vi "FSF_Query.vi"(0 "System no.":i32=1 min=1 max=4 step=1, 2 "Axes to query":string[](array[string]), 3 "All axes?":bool, 4 "Axis identifier?":bool, 5 "error in":errorcluster) -> (14 "Force value 1":dbl[](array[numeric]) format="%.6f", 15 "Position offset":dbl[](array[numeric]) format="%.6f", 16 "Force value 2":dbl[](array[numeric]) format="%.6f", 19 "error out":errorcluster)   [LabVIEW 2020]
doc: "Returns parameters used for last find surface procedure (FSF).\n\nC-413:"
panel:
  # "Returns the parameters set by FSF."
  # "If all axes: use"
  # "Query"
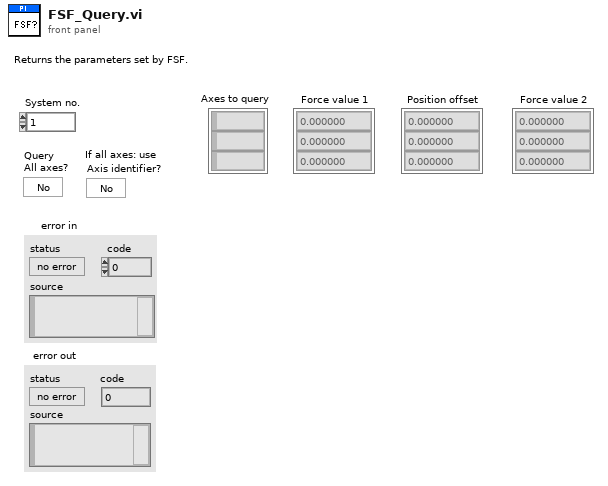
[diagram p1: front panel]
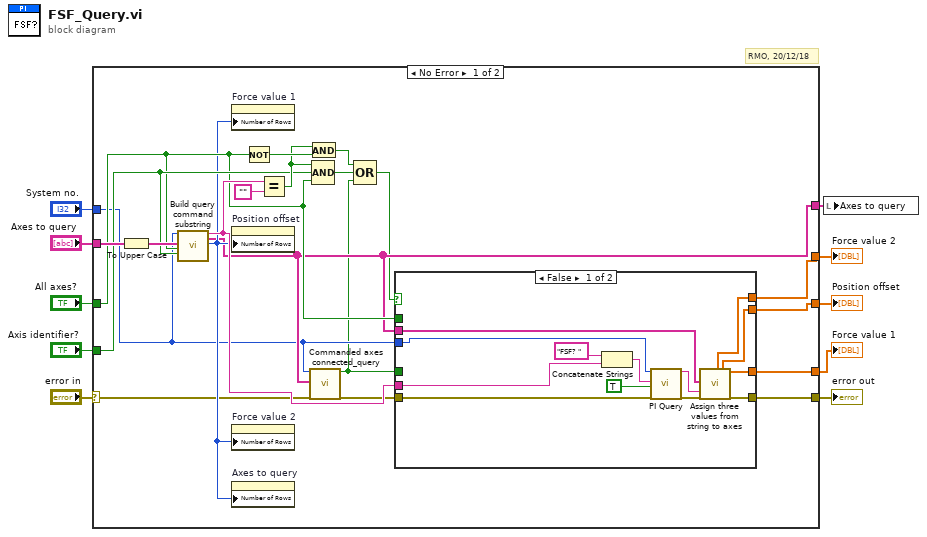
[diagram p0: block diagram]
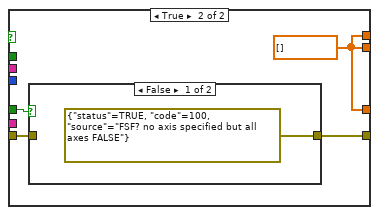
[diagram p2: hidden frame]
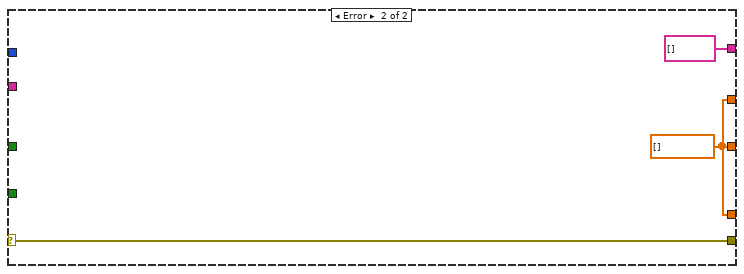
[diagram p4: hidden frame]
diagram:
  # "RMO, 20/12/18"
  n1 = case shown="No Error" "error in" {
    selector: "error in" -> [w11 w51]
    tunnel: [w31 w52] -> w10
    tunnel: "Axes to query" -> [w30 _]
    tunnel: [w22 w51] -> w8
    tunnel: "System no." -> [w16 _]
    tunnel: [w17 string[] [] ("Axes to query out")] -> w6
    tunnel: "Axis identifier?" -> [w24 _]
    tunnel: "All axes?" -> [w23 _]
    tunnel: [w21 w52] -> w3
    tunnel: [w20 w52] -> w2
    frame No Error {
      n2 = To Upper Case(1:w30) -> (0:w28:string[])
      n3 = call "Build query command substring.vi"("System no."=w16, "Axes to query in"=w28, "Query\nAll axes?"=w23, "For all axes: use\nAxis identifier?"=w24) -> ("Command substring"=w27:string, "Axes to query out"=w17:string[], "Number of rows"=w19:u32)  [unwired: 2 in, 11 out]
      n4 = property on="Force value 1" class="Arr (strict)"("Number of Rows"=w19) -> ()  [unwired: 2 in, 2 out]
      n5 = property on="Position offset" class="Arr (strict)"("Number of Rows"=w19) -> ()  [unwired: 2 in, 2 out]
      n6 = property on="Force value 2" class="Arr (strict)"("Number of Rows"=w19) -> ()  [unwired: 2 in, 2 out]
      n7 = property on="Axes to query" class="Arr (strict)"("Number of Rows"=w19) -> ()  [unwired: 2 in, 2 out]
      n8 = Not(x=w23) -> (.not. x?=w26:bool)
      n9 = Equal?(x=w27, y="" ("x")) -> (x = y?=w25:bool)
      n10 = And(x=w25, y=w26) -> (x .and. y?=w15:bool)
      n11 = call "Commanded axes connected_query.vi"("System no."=w16, "Commanded axes"=w17, "error in"=w11) -> ("Controller error"=w12:bool, "error out"=w18:errorcluster)  [unwired: 1 in, 14 out]
      n12 = Compound Arithmetic op=AND(w25, w24, w23) -> (w14:bool)
      n13 = Compound Arithmetic op=OR(w15, w14, w12) -> (w13:bool)
      n14 = case shown="False" w13 {
        tunnel: [w37 w47] -> w31
        tunnel: w18 -> [w34 w46]
        tunnel: w27 -> [w41 _]
        tunnel: w16 -> [w40 _]
        tunnel: w17 -> [w39 _]
        tunnel: w23 -> [_ _]
        tunnel: [w38 w48] -> w22
        tunnel: [w36 w47] -> w21
        tunnel: [w35 w47] -> w20
        tunnel: w12 -> [_ w45]
        frame False {
          n15 = Concatenate Strings("FSF? ", w41) -> (w42:string)
          n16 = call "PI Query.vi"("System no."=w40, "String to send"=w42, "Attach termination char.?"=TRUE ("Attach Linefeed?"), "error in"=w34) -> ("String read"=w32:string, "error out"=w33:errorcluster)  [unwired: 3 in, 11 out]
          n17 = call "Assign three values from string to axes.vi"("Queried axes"=w39, "Input String"=w32, "error in"=w33) -> ("Values 3"=w35:dbl[], "Values 2"=w36:dbl[], "Values 1"=w37:dbl[], "error out"=w38:errorcluster)  [unwired: 13 out]
        }
        frame True {
          w47 = dbl[] [] ("Values")
          n18 = case shown="False" w45 {
            tunnel: [errorcluster {"status"=TRUE, "code"=100, "source"="FSF? no axis specified but all axes FALSE"} ("error out") w50] -> w48
            tunnel: w46 -> [_ w50]
            frame False {
            }
            frame True {
            }
          }
        }
      }
    }
    frame Error {
      w52 = dbl[] [] ("Values")
    }
  }
  "error out" <- w8
  "Force value 1" <- w10
  "Force value 2" <- w2
  "Position offset" <- w3
  n19 = local write "Axes to query"(w6) -> ()
